vi "New Connection DVR.vi"(8 "error in (no error)":errorcluster, 11 "Connection in":refnum<class "Connection.lvclass">) -> (0 "error out":errorcluster, 3 "Connection DVR out":refnum<data-value>)   [LabVIEW 2010, in "MDSplus.lvlib" / "Connection.lvclass"]
uses:
  <vilib>/MDSplus/Classes/Connection_Class/Connection.lvclass
  <vilib>/MDSplus/Classes/Connection_Class/Connection.lvclass/Connection.ctl
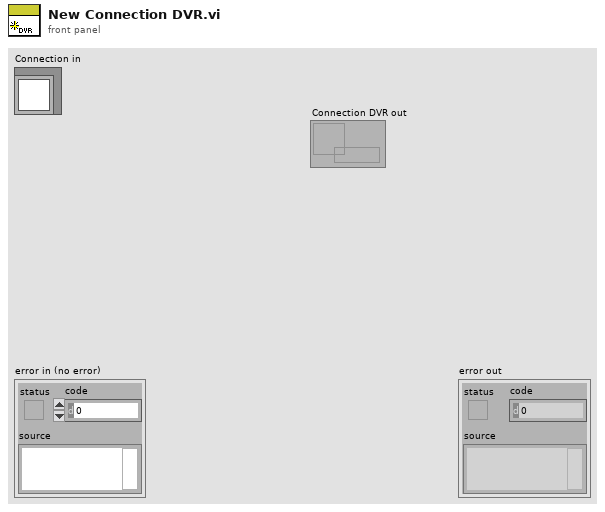
[diagram p1: front panel]
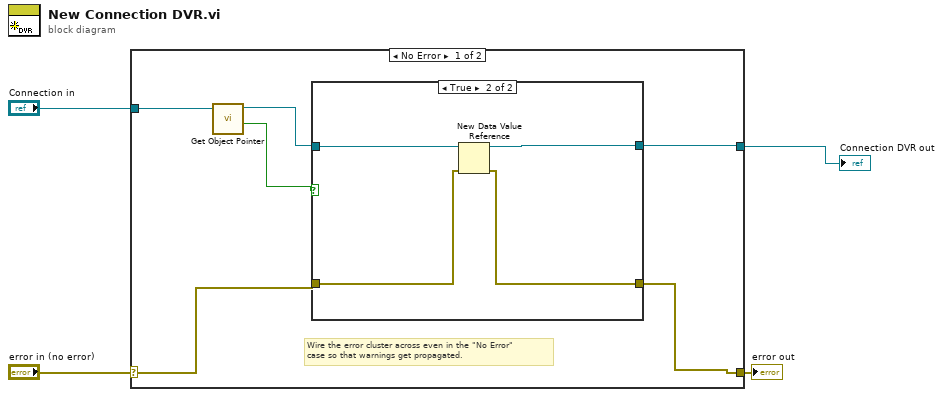
[diagram p0: block diagram]
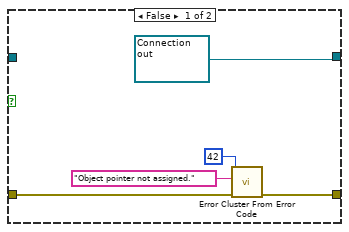
[diagram p2: hidden frame]
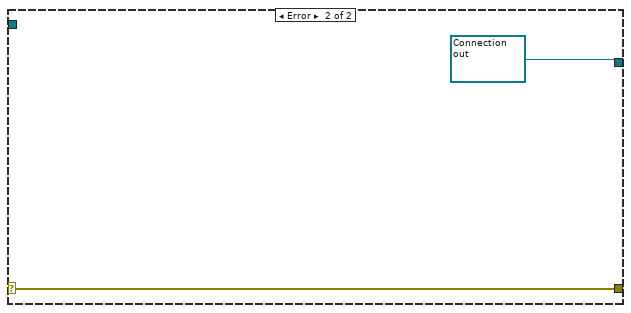
[diagram p3: hidden frame]
diagram:
  n1 = case shown="No Error" "error in (no error)" {
    selector: "error in (no error)" -> [w8 w21]
    tunnel: [w7 w21] -> w3
    tunnel: "Connection in" -> [w10 _]
    tunnel: [w6 refnum<data-value> refnum ("data value reference 2")] -> w1
    frame No Error {
      # "Wire the error cluster across even in the \"No Error\"\ncase so that warnings get propagated."
      n2 = call <vilib>:"Get Object Pointer.vi"("Connection in"=w10) -> ("Assigned object pointer?"=w5:bool, "Connection out"=w9:refnum<class "Connection.lvclass">)  [unwired: 7 in, 2 out]
      n3 = case shown="True" w5 {
        tunnel: w8 -> [w13 w19]
        tunnel: [w12 w17] -> w7
        tunnel: w9 -> [_ w18]
        tunnel: [refnum<data-value> refnum ("data value reference 2") w16] -> w6
        frame False {
          n4 = call <vilib>:"Error Cluster From Error Code.vi"("error in (no error)"=w13, "error message (\"\")"="Object pointer not assigned." ("error message (\"\")"), "error code (0)"=42) -> ("error out"=w12:errorcluster)  [unwired: 6 in]
        }
        frame True {
          n5 = New Data Value Reference(data value=w18, error in=w19) -> (data value reference=w16:refnum<data-value>, error out=w17:errorcluster)
        }
      }
    }
    frame Error {
    }
  }
  "error out" <- w3
  "Connection DVR out" <- w1
